vi "LVClass_HasoData Write HasoData.vi"(8 "error in (no error)":errorcluster, 10 "HasoData":T1, 11 "HasoData in":refnum<class "HasoData.lvclass">) -> (0 "error out":errorcluster, 3 "HasoData out":refnum<class "HasoData.lvclass">)   [LabVIEW 2020, in "HasoData.lvclass"]
uses:
  HasoData.lvclass
  Controls/ClassID.ctl
  Controls/Handle creation.ctl
  HasoData.lvclass/HasoData.ctl
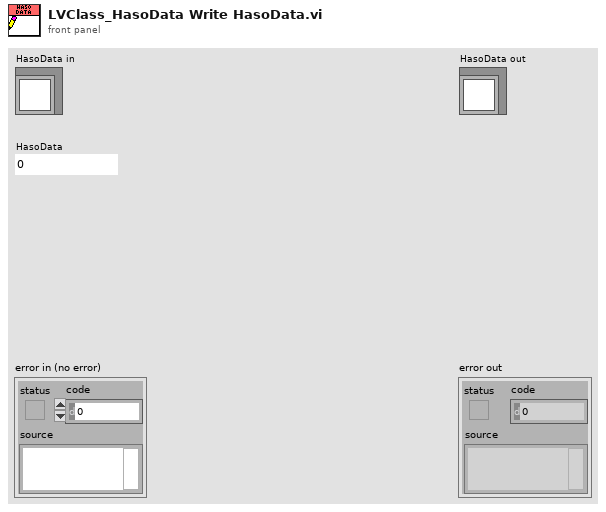
[diagram p1: front panel]
types:
  T1 = typedef "ClassID.ctl" = i64
  T2 = typedef "Handle creation.ctl" = enum16{"By ctor", "By write function"}
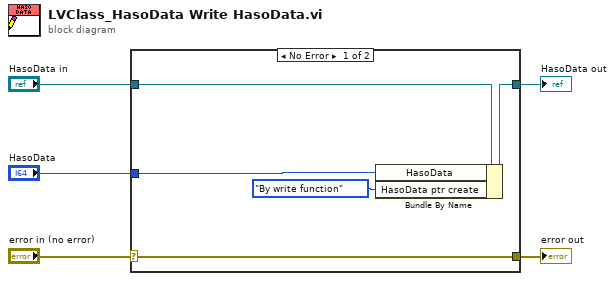
[diagram p0: block diagram]
diagram:
  n1 = case shown="No Error" "error in (no error)" {
    selector: "error in (no error)" -> [w10 w11]
    tunnel: [w10 w11] -> w4
    tunnel: [w8 w12] -> w2
    tunnel: "HasoData in" -> [w9 w12]
    tunnel: "HasoData" -> [w7 _]
    frame No Error {
      n2 = Bundle By Name(cluster=w9, "HasoData"=w7, "HasoData ptr create"=Handle_creation."By write function") -> (w8:refnum<class "HasoData.lvclass">)
    }
    frame Error {
    }
  }
  "error out" <- w4
  "HasoData out" <- w2
